vi "FPGAcode4_Debug.vi"(7 "Speed Bracket":i32, 8 "Thresholds in":i32[](array[numeric])=[0, 0, 0, 0, 0, 0, 0, 0, 0, 0, 0], 9 "Clock Speed (Hz)":i32=40000000, 10 "Calibrate":bool=TRUE, 11 "Detector Waveform In":sgl[][](array[numeric])) -> (0 "Thresholds out":i32[](array[numeric]), 1 "Charge":fxp<+,32,-41>[](array[numeric]), 2 "Mass":fxp<+/-,64,-19>[](array[numeric]), 3 "PSU Response":bool[](array[boolean]), 4 "Velocity Count":i32[](array[numeric]), 5 "Max Stop Point":T1)   [LabVIEW 2015]
uses:
  FPGA3/Limits_In.ctl
  FPGA3/Detector_Cluster.ctl
  FPGA3/Correlations.ctl
panel:
  in  "User Trigger?":bool
  in  "User Trigger Distance":fxp<+/-,34,18> format="%.3g"
  out "User Trigger":bool
  in  "Boxcar 3 Size Factor":fxp<+/-,32,16>=0.199951171875 format="%.2g"
  in  "Charge Error Factor":fxp<+/-,32,16>=1.499969482421875 format="%.2g"
  in  "Max Correlation Factor":fxp<+,32,4>=1.1000000052154064 format="%.3g"
  in  "Threshold Factor":fxp<+/-,32,16>=1.299957275390625 format="%.2g"
  out "DCS 2":bool
  out "DCS 1":bool
  in  "Limits":T2={"High Charge Limit"=4.54747350780585e-13, "Low Charge Limit"=0.0, "High Velocity Limit"=262143.0, "Low Velocity Limit"=0.0, "High Mass Limit"=7.27595761248936e-12, "Low Mass Limit"=0.0, "High Voltage"=2200000.0}
  in  "Armed":bool
  out "Plates":bool
  in  "One Shot":bool
  # "These factors above are in the front\npanel so it is possible to experiment\nwith many different configurations\nof the FPGA on the fly. One can even\nchange the relative size of one filter."
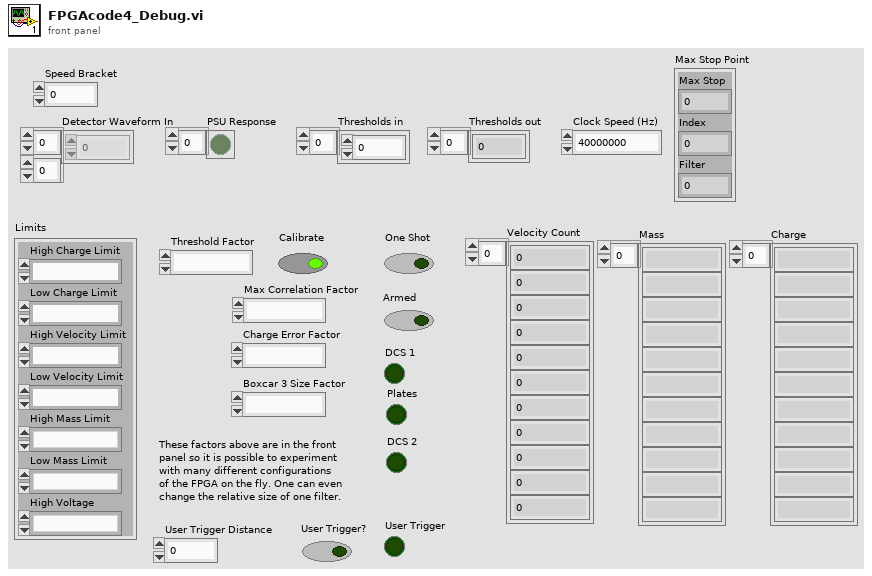
[diagram p1: front panel]
types:
  T1 = cluster{"Max Stop":u8, "Index":i32, "Filter":i32}
  T2 = typedef "Limits_In.ctl" = cluster{"High Charge Limit":fxp<+,32,-41>, "Low Charge Limit":fxp<+,32,-41>, "High Velocity Limit":fxp<+,18,18>, "Low Velocity Limit":fxp<+,18,18>, "High Mass Limit":fxp<+/-,33,-36>, "Low Mass Limit":fxp<+/-,33,-36>, "High Voltage":fxp<+,16,22>}
  T3 = cluster{i32, fxp<+/-,64,-19>, "High Charge Limit":fxp<+,32,-41>}[]
  T4 = typedef "Detector_Cluster.ctl" = cluster{"Det 1":i32, "Det 2":i32}
  T5 = cluster{"Filter 1":T4, "Filter 2":T4, "Filter 3":T4, "Filter 4":T4}
  T6 = cluster{"Distance to PSU":fxp<+/-,32,5>, "Distance to end of PSU":fxp<+/-,32,5>, "Distance to DCS 2":fxp<+/-,32,5>, "Distance to DCS 1":fxp<+/-,32,5>, "Distance to front of LEIL Chamber":fxp<+/-,32,5>}
  T7 = cluster{"Detector Max Speed Count":i32, "Detector Min Speed Count":i32, "Gap Max Speed Count":i32, "Gap Min Speed Count":i32}
  T8 = cluster{"Distance to PSU":fxp<+/-,64,37>, "Distance to end of PSU":fxp<+/-,64,37>, "Distance to DCS 2":fxp<+/-,64,37>, "Distance to DCS 1":fxp<+/-,64,37>, "Distance to front of LEIL Chamber":fxp<+/-,64,37>}
  T9 = cluster{"Filter 1":T4, "Filter 2":T4, "Filter 3":T4, "Filter 4":T4}[]
  T10 = cluster{"First Detector Count":i32, "Detector Gap Count":i32, "Second Detector Count":i32, "Second Detector Final Count":i32}
  T11 = typedef "Correlations.ctl" = cluster{"First Correlation":i32, "Latest Correlation":i32}
  T12 = cluster{cluster{i16, i16}, cluster{"Det 1":i16, "Det 2":i16}, cluster{"Det 1":i16, "Det 2":i16}, cluster{"Det 1":i16, "Det 2":i16}}
  T13 = cluster{cluster{"Det 1":i16, "Det 2":i16}, cluster{"Det 1":i16, "Det 2":i16}, cluster{"Det 1":i16, "Det 2":i16}, cluster{"Det 1":i16, "Det 2":i16}}
  T14 = cluster{"Distance to PSU":fxp<+/-,64,69>, "Distance to end of PSU":fxp<+/-,64,69>, "Distance to DCS 2":fxp<+/-,64,69>, "Distance to DCS 1":fxp<+/-,64,69>, "Distance to front of LEIL Chamber":fxp<+/-,64,69>}
  T15 = cluster{"Distance to PSU":i32, "Distance to end of PSU":i32, "Distance to DCS 2":i32, "Distance to DCS 1":i32, "Distance to front of LEIL Chamber":i32}
  T16 = cluster{i32, fxp<+/-,64,-19>, "High Charge Limit":fxp<+,32,-41>}
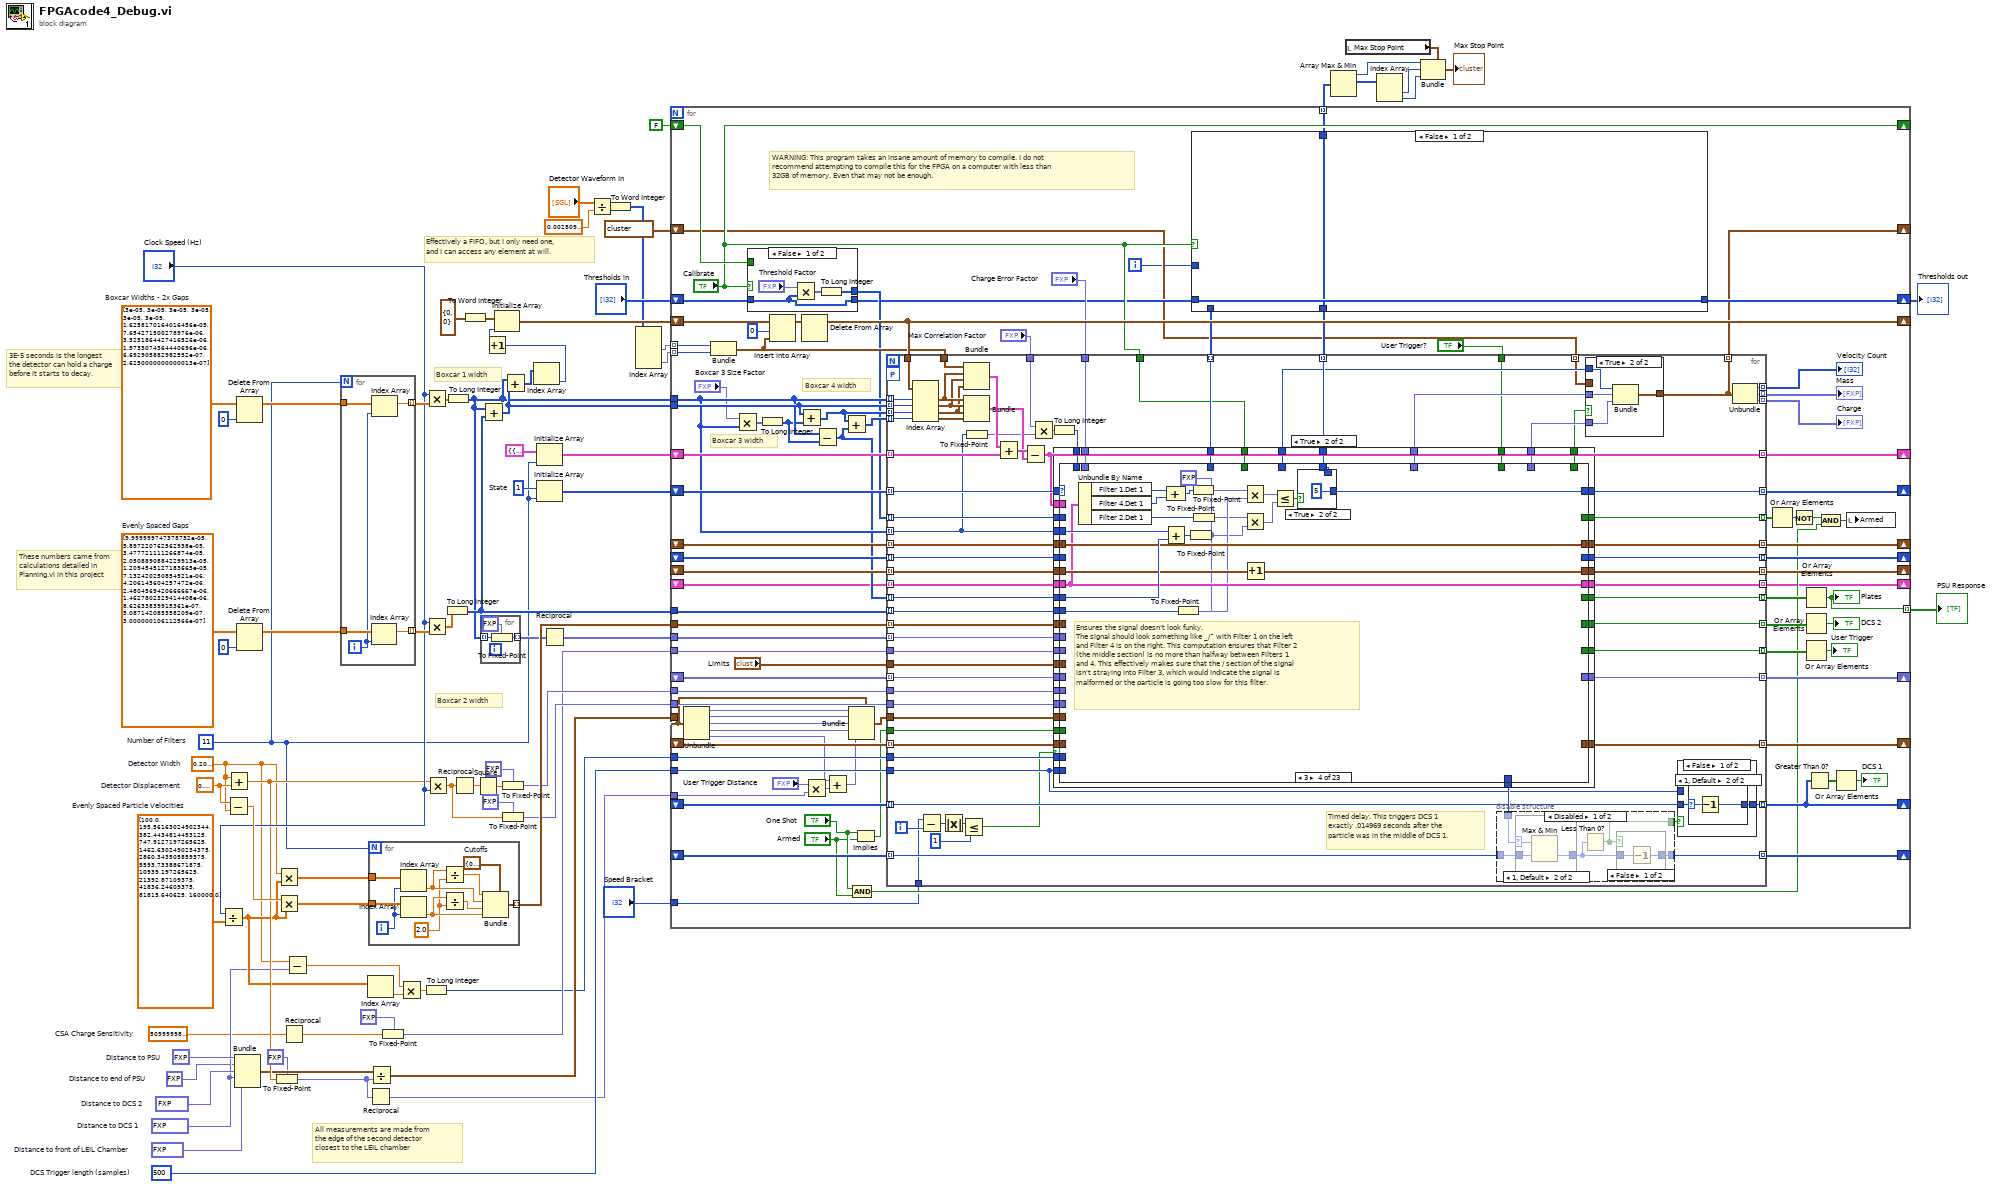
[diagram p0: block diagram]
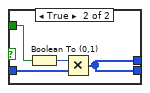
[diagram p2: hidden frame]
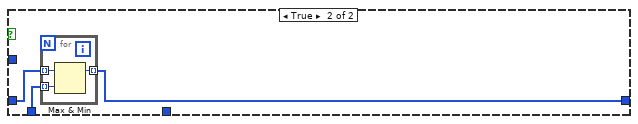
[diagram p3: hidden frame]
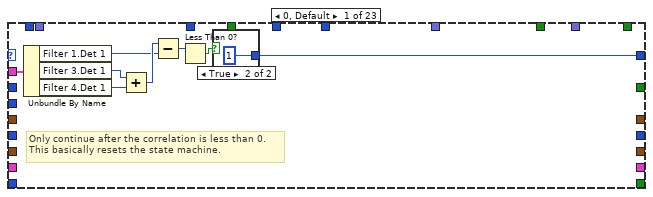
[diagram p5: hidden frame]
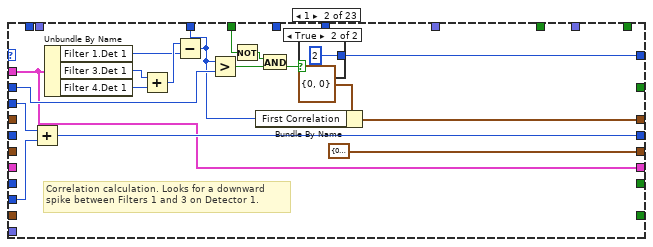
[diagram p7: hidden frame]
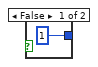
[diagram p8: hidden frame]
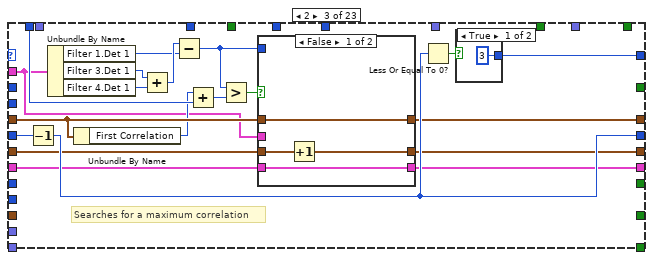
[diagram p9: hidden frame]
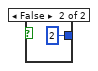
[diagram p10: hidden frame]
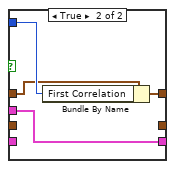
[diagram p11: hidden frame]
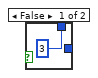
[diagram p12: hidden frame]
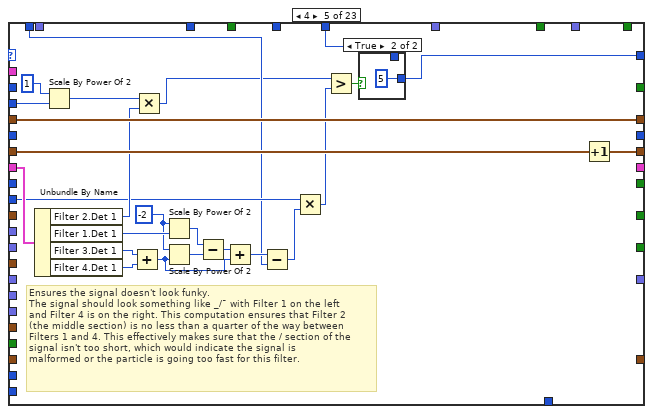
[diagram p13: hidden frame]
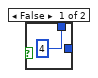
[diagram p14: hidden frame]
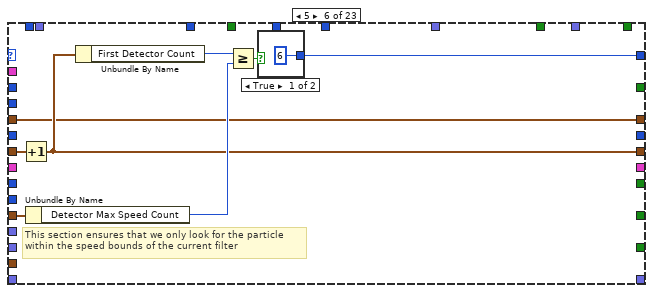
[diagram p15: hidden frame]
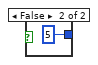
[diagram p16: hidden frame]
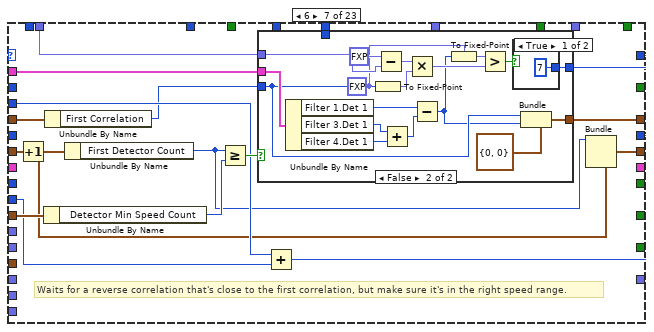
[diagram p17: hidden frame]
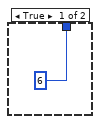
[diagram p18: hidden frame]
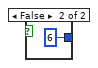
[diagram p19: hidden frame]
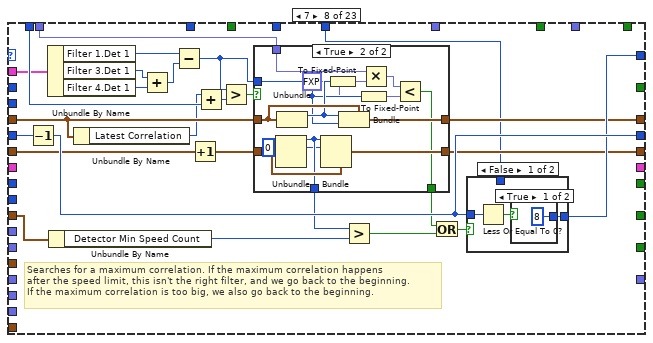
[diagram p20: hidden frame]
diagram:
  w10 = dbl[] [3e-05, 3e-05, 3e-05, 3e-05, 3e-05, 3e-05, 1.6258170164016456e-05, 7.654271500278976e-06, 3.5251864427416526e-06, 1.5733074364440696e-06, 6.692905882982552e-07, 2.6250000000000013e-07]  # Boxcar Widths - 2x Gaps
  w28 = fxp<+/-,32,5> 4.297679997980595  # Distance to front of LEIL Chamber
  w34 = u16 500  # DCS Trigger length (samples)
  w39 = fxp<+/-,32,5> -1.3589000031352043  # Distance to DCS 1
  w42 = fxp<+/-,32,5> 2.6162000000476837  # Distance to DCS 2
  w31 = fxp<+/-,32,5> 2.0  # Distance to end of PSU
  w43 = fxp<+/-,32,5> 1.1000000014901161  # Distance to PSU
  w27 = sgl 5100000000000000.0  # CSA Charge Sensitivity
  w74 = u8 1  # State
  w40 = sgl 0.6  # Detector Displacement
  w78 = sgl[] [0.0001, 5.8972208e-05, 3.477721e-05, 2.050889e-05, 1.2094545e-05, 7.1324203e-06, 4.2061456e-06, 2.480457e-06, 1.4627802e-06, 8.6263384e-07, 5.087142e-07, 3e-07]  # Evenly Spaced Gaps
  w59 = sgl[] [100.0, 195.56163, 382.44348, 747.9127, 1462.6302, 2860.3435, 5593.734, 10939.197, 21392.871, 41836.246, 81815.64, 160000.0]  # Evenly Spaced Particle Velocities
  w35 = sgl 0.21  # Detector Width
  w32 = 11  # Number of Filters
  # "All measurements are made from\nthe edge of the second detector\nclosest to the LEIL chamber"
  # "Effectively a FIFO, but I only need one,\nand I can access any element at will."
  # "Boxcar 2 width"
  # "Boxcar 1 width"
  # "3E-5 seconds is the longest\nthe detector can hold a charge\nbefore it starts to decay."
  # "These numbers came from\ncalculations detailed in\nPlanning.vi in this project"
  n1 = Divide(x="Clock Speed (Hz)", y=w59) -> (x/y=w41:sgl[])
  n2 = Subtract(x=w40, y=w35) -> (x-y=w58:sgl)
  n3 = Add(x=w35, y=w40) -> (x+y=w46:sgl)
  n4 = Bundle("Distance to PSU"=w43, "Distance to end of PSU"=w31, "Distance to DCS 2"=w42, "Distance to DCS 1"=w39, "Distance to front of LEIL Chamber"=w28) -> (w45:T6)  [unwired: 1 in]
  n5 = Delete From Array(array=w10, index=0) -> (array with subset deleted=w67:dbl[])  [unwired: 1 in, 1 out]
  n6 = Delete From Array(array=w78, index=0) -> (array with subset deleted=w69:sgl[])  [unwired: 1 in, 1 out]
  n7 = To Fixed-Point(fixed-point type=fxp<+/-,32,1> 0.0, number=w46) -> (fixed-point=w30:fxp<+/-,32,1>)
  n8 = Multiply(x=w35, y=w41) -> (x*y=w76:sgl[])
  n9 = Multiply(x=w58, y=w41) -> (x*y=w77:sgl[])
  n10 = Reciprocal(x=w27) -> (1/x=w48:sgl)
  n11 = Subtract(x=w35, y=w39) -> (x-y=w37:sgl)
  n12 = for {
    N: w32 -> [_]
    tunnel: w69 -> [w86]
    tunnel: [w83] -> w68 mode=indexing
    tunnel: w67 -> [w85]
    tunnel: [w84] -> w66 mode=indexing
    i -> [w82]
    n13 = Index Array(array=w86, index=w82) -> (element=w83:sgl)
    n14 = Index Array(array=w85, index=w82) -> (element=w84:dbl)
  }
  n15 = Index Array(array=w41) -> (element=w38:sgl)  [unwired: 1 in]
  n16 = Reciprocal(x=w30) -> (1/x=w29:fxp<+/-,34,33>)
  n17 = for {
    N: w32 -> [_]
    tunnel: w77 -> [w96]
    tunnel: w76 -> [w95]
    tunnel: [w94] -> w71 mode=indexing
    i -> [w93]
    w87 = sgl 2.0 ("y")
    w92 = T7 {"Detector Max Speed Count"=0, "Detector Min Speed Count"=0, "Gap Max Speed Count"=0, "Gap Min Speed Count"=0}  # Cutoffs
    n18 = Index Array(array=w95, index=w93) -> (element=w91:sgl)
    n19 = Index Array(array=w96, index=w93) -> (element=w88:sgl)
    n20 = Divide(x=w91, y=w87) -> (x/y=w90:sgl)
    n21 = Divide(x=w88, y=w87) -> (x/y=w89:sgl)
    n22 = Bundle(cluster=w92, "Detector Max Speed Count"=w90, "Detector Min Speed Count"=w91, "Gap Max Speed Count"=w89, "Gap Min Speed Count"=w88) -> (w94:T7)
  }
  n23 = Divide(x=w45, y=w30) -> (x/y=w44:T8)
  n24 = To Fixed-Point(fixed-point type=fxp<+,32,-51> 0.0, number=w48) -> (fixed-point=w47:fxp<+,32,-51>)
  n25 = Multiply(x=w37, y=w38) -> (x*y=w36:sgl)
  n26 = To Long Integer(number=w36) -> (32bit integer=w33:i32)
  n27 = Multiply(x="Clock Speed (Hz)", y=w66) -> (x*y=w70:dbl[])
  n28 = Multiply(x="Clock Speed (Hz)", y=w68) -> (x*y=w75:sgl[])
  n29 = Multiply(x=w46, y="Clock Speed (Hz)") -> (x*y=w51:sgl)
  n30 = To Long Integer(number=w75) -> (32bit integer=w65:i32[])
  n31 = To Long Integer(number=w70) -> (32bit integer=w22:i32[])
  n32 = Reciprocal(x=w51) -> (1/x=w55:sgl)
  n33 = To Word Integer(number=T4 {"Det 1"=0, "Det 2"=0} ("Detectors")) -> (16bit integer=w64:cluster{"Det 1":i16, "Det 2":i16})
  n34 = Square(x=w55) -> (x^2=w54:sgl)
  n35 = Add(x=w22, y=w65) -> (x+y=w23:i32[])
  n36 = for {
    tunnel: w22 -> [w99] mode=indexing
    tunnel: [w98] -> w61 mode=indexing
    n37 = To Fixed-Point(fixed-point type=fxp<+/-,32,32> 0.0, number=w99) -> (fixed-point=w98:fxp<+/-,32,32>)
  }
  n38 = To Fixed-Point(fixed-point type=fxp<+/-,32,-42> 0.0, number=w54) -> (fixed-point=w57:fxp<+/-,32,-42>)
  n39 = To Fixed-Point(fixed-point type=fxp<+,32,28> 0.0, number=w51) -> (fixed-point=w49:fxp<+,32,28>)
  n40 = Add(x=w22, y=w23) -> (x+y=w21:i32[])
  n41 = Index Array(array=w21) -> (element=w20:i32)  [unwired: 1 in]
  n42 = Increment(x=w20) -> (x+1=w19:i32)
  n43 = Initialize Array(w64, w19) -> (w81:cluster{"Det 1":i16, "Det 2":i16}[])
  n44 = Initialize Array(T5 {"Filter 1"={"Det 1"=0, "Det 2"=0}, "Filter 2"={"Det 1"=0, "Det 2"=0}, "Filter 3"={"Det 1"=0, "Det 2"=0}, "Filter 4"={"Det 1"=0, "Det 2"=0}} ("cluster"), w32) -> (w72:T9)
  n45 = Initialize Array(w74, w32) -> (w73:u8[])
  n46 = Reciprocal(x=w61) -> (1/x=w60:fxp<+/-,34,2>[])
  n47 = Divide(x="Detector Waveform In", y=sgl 0.00281) -> (x/y=w26:sgl[][])
  n48 = To Word Integer(number=w26) -> (16bit integer=w12:i16[][])
  n49 = Index Array(array=w12) -> (element #1=w14:i16[], element #2=w13:i16[])  [unwired: 4 in]
  n50 = for {
    shift-right: [w188] -> _
    shift-left: w81 -> [w189]
    shift-right: [w187] -> _
    shift-left: w72 -> [w180]
    shift-right: [w185] -> _
    shift-left: w73 -> [w186]
    shift-right: [w184] -> _
    shift-left: _ -> [w183]
    shift-right: [w182] -> _
    shift-left: _ -> [w181]
    tunnel: w71 -> [w179]
    shift-right: [w178] -> _
    shift-left: _ -> [w177]
    tunnel: w22 -> [w174]
    tunnel: w23 -> [w176]
    tunnel: w65 -> [w175]
    tunnel: w60 -> [w173]
    shift-right: [w172] -> _
    shift-left: _ -> [w171]
    tunnel: w57 -> [w170]
    tunnel: w47 -> [w169]
    tunnel: w49 -> [w168]
    tunnel: w44 -> [w155]
    shift-right: [w167] -> _
    shift-left: _ -> [w166]
    shift-right: [w165] -> w24
    shift-left: "Thresholds in" -> [w164]
    shift-right: ["Calibrate"] -> _
    shift-left: FALSE ("Calibrate") -> [w163]
    tunnel: w34 -> [w162]
    tunnel: w33 -> [w161]
    shift-right: [w159] -> _
    shift-left: _ -> [w160]
    shift-right: [w158] -> _
    shift-left: _ -> [w157]
    tunnel: w29 -> [w156]
    shift-right: [w107] -> _
    shift-left: T3 [{0, 0.0, "High Charge Limit"=0.0}, {0, 0.0, "High Charge Limit"=0.0}, {0, 0.0, "High Charge Limit"=0.0}, {0, 0.0, "High Charge Limit"=0.0}, {0, 0.0, "High Charge Limit"=0.0}, {0, 0.0, "High Charge Limit"=0.0}, {0, 0.0, "High Charge Limit"=0.0}, {0, 0.0, "High Charge Limit"=0.0}, {0, 0.0, "High Charge Limit"=0.0}, {0, 0.0, "High Charge Limit"=0.0}, {0, 0.0, "High Charge Limit"=0.0}] -> [w106]
    tunnel: [w115] -> w9 mode=indexing
    shift-right: [w114] -> _
    shift-left: _ -> [w113]
    tunnel: w14 -> [w112] mode=indexing
    tunnel: w13 -> [w111] mode=indexing
    tunnel: [w102] -> w8 mode=indexing
    tunnel: "Speed Bracket" -> [w100]
    i -> [w101]
    # "WARNING: This program takes an insane amount of memory to compile. I do not\nrecommend attempting to compile this for the FPGA on a computer with less than\n32GB of memory. Even that may not be enough."
    # "Boxcar 3 width"
    # "Boxcar 4 width"
    n51 = Unbundle(w155) -> ("Distance to PSU"=w137:fxp<+/-,64,37>, "Distance to end of PSU"=w136:fxp<+/-,64,37>, "Distance to DCS 2"=w135:fxp<+/-,64,37>, "Distance to DCS 1"=w132:fxp<+/-,64,37>, "Distance to front of LEIL Chamber"=w131:fxp<+/-,64,37>)
    n52 = Bundle(w112, w111) -> (w116:cluster{i16, i16})  [unwired: 1 in]
    n53 = Multiply(x="Boxcar 3 Size Factor", y=w174) -> (x*y=w150:fxp<+/-,64,48>[])
    n54 = case shown="False" "Calibrate" {
      tunnel: w164 -> [w191 w197]
      tunnel: [w191 w194] -> w108
      tunnel: w163 -> [_ w196]
      tunnel: [w190 w194] -> w109
      frame False {
        n55 = Multiply(x="Threshold Factor", y=w191) -> (x*y=w192:fxp<+/-,64,48>[])
        n56 = To Long Integer(number=w192) -> (32bit integer=w190:i32[])
      }
      frame True {
        n57 = Boolean To (0,1)(Boolean=w196) -> (0, 1=w195:i16)
        n58 = Multiply(x=w195, y=w197) -> (x*y=w194:i32[])
      }
    }
    n59 = To Long Integer(number=w150) -> (32bit integer=w151:i32[])
    n60 = Insert Into Array(array=w189, index=0, new element=w116) -> (w154:cluster{"Det 1":i16, "Det 2":i16}[])
    n61 = Add(x=w176, y=w151) -> (x+y=w148:i32[])
    n62 = Delete From Array(array=w154) -> (array with subset deleted=w188:cluster{"Det 1":i16, "Det 2":i16}[])  [unwired: 2 in, 1 out]
    n63 = Multiply(x="User Trigger Distance", y=w156) -> (x*y=w133:fxp<+/-,64,49>)
    n64 = Subtract(x=w174, y=w151) -> (x-y=w146:i32[])
    n65 = Add(x=w131, y=w133) -> (x+y=w130:fxp<+/-,64,50>)
    n66 = Add(x=w148, y=w146) -> (x+y=w147:i32[])
    n67 = Bundle(cluster=w155, "Distance to PSU"=w137, "Distance to end of PSU"=w136, "Distance to DCS 2"=w135, "Distance to DCS 1"=w132, "Distance to front of LEIL Chamber"=w130) -> (w134:T8)
    n68 = And(x="One Shot", y="Armed") -> (x .and. y?=w121:bool)
    n69 = Implies(1:"Armed", 2:"One Shot") -> (0:w141:bool)
    n70 = for {
      tunnel: w188 -> [w282]
      tunnel: [w265] -> w187 mode=indexing
      tunnel: w186 -> [w281] mode=indexing
      tunnel: [w279] -> w185 mode=indexing
      tunnel: w109 -> [w280] mode=indexing
      tunnel: [w278] -> w184 mode=indexing
      tunnel: w183 -> [w277] mode=indexing
      tunnel: [w276] -> w182 mode=indexing
      tunnel: w181 -> [w275] mode=indexing
      tunnel: w180 -> [w269] mode=indexing
      tunnel: w116 -> [w274]
      tunnel: w179 -> [w264] mode=indexing
      tunnel: [w263] -> w178 mode=indexing
      tunnel: w177 -> [w262] mode=indexing
      tunnel: w174 -> [w261] mode=indexing
      tunnel: w176 -> [w260] mode=indexing
      tunnel: w148 -> [w259] mode=indexing
      tunnel: w147 -> [w258] mode=indexing
      tunnel: w174 -> [w207] mode=indexing
      tunnel: "Max Correlation Factor" -> [w257]
      tunnel: w146 -> [w256] mode=indexing
      tunnel: w175 -> [w206] mode=indexing
      tunnel: "Charge Error Factor" -> [w255]
      tunnel: [w254] -> w143 mode=indexing
      tunnel: w173 -> [w253] mode=indexing
      tunnel: "Limits" -> [w252]
      tunnel: [w251] -> w172 mode=indexing
      tunnel: w171 -> [w250] mode=indexing
      tunnel: w170 -> [w249]
      tunnel: w169 -> [w248]
      tunnel: w168 -> [w247]
      tunnel: w134 -> [w246]
      tunnel: [w245] -> w167 mode=indexing
      tunnel: w166 -> [w244] mode=indexing
      tunnel: [w243] -> w142 mode=indexing
      tunnel: w141 -> [w242]
      tunnel: w162 -> [w239]
      tunnel: w161 -> [w241]
      tunnel: [w238] -> w159 mode=indexing
      tunnel: w160 -> [w237] mode=indexing
      tunnel: [w235] -> w158 mode=indexing
      tunnel: w157 -> [w234] mode=indexing
      tunnel: [w233] -> w129 mode=indexing
      tunnel: [w232] -> w128 mode=indexing
      tunnel: [w231] -> w127 mode=indexing
      tunnel: [w230] -> w124 mode=indexing
      tunnel: "User Trigger?" -> [w223]
      tunnel: w113 -> [w220] mode=indexing
      tunnel: [w219] -> w114 mode=indexing
      tunnel: "Calibrate" -> [w217]
      tunnel: [w215] -> w107 mode=indexing
      tunnel: w106 -> [w216] mode=indexing
      tunnel: [w214] -> w105 mode=indexing
      tunnel: [w213] -> w104 mode=indexing
      tunnel: [w212] -> w103 mode=indexing
      workers-P: _ -> [_]
      tunnel: w100 -> [w211]
      i -> [w222]
      # "Timed delay. This triggers DCS 1\nexactly .014969 seconds after the\nparticle was in the middle of DCS 1."
      n71 = Index Array(array=w282, index #1=w261, index #2=w260, index #3=w259, index #4=w258) -> (element #1=w272:cluster{"Det 1":i16, "Det 2":i16}, element #2=w271:cluster{"Det 1":i16, "Det 2":i16}, element #3=w270:cluster{"Det 1":i16, "Det 2":i16}, element #4=w273:cluster{"Det 1":i16, "Det 2":i16})
      n72 = Subtract(x=w211, y=w222) -> (x-y=w221:i32)
      n73 = Absolute Value(x=w221) -> (abs(x)=w210:i32)
      n74 = Less Or Equal?(x=w210, y=1) -> (x <= y?=w209:bool)
      n75 = Bundle(w274, w272, w271, w270) -> (w268:T12)  [unwired: 1 in]
      n76 = Bundle(w272, w271, w270, w273) -> (w266:T13)  [unwired: 1 in]
      n77 = To Fixed-Point(number=w207) -> (fixed-point=w225:fxp<+/-,32,32>)  [unwired: 1 in]
      n78 = Add(x=w268, y=w269) -> (x+y=w267:T5)
      n79 = Subtract(x=w267, y=w266) -> (x-y=w265:T5)
      n80 = Multiply(x=w257, y=w225) -> (x*y=w226:fxp<+/-,64,36>)
      n81 = To Long Integer(number=w226) -> (32bit integer=w224:i32)
      n82 = case shown="True" w209 {
        tunnel: w281 -> [_ w326]
        tunnel: w280 -> [_ w325]
        tunnel: [_ w324] -> w279
        tunnel: [_ w323] -> w278
        tunnel: w277 -> [_ w322]
        tunnel: [_ w321] -> w276
        tunnel: w275 -> [_ w320]
        tunnel: w265 -> [_ w319]
        tunnel: w264 -> [_ w318]
        tunnel: [_ w317] -> w263
        tunnel: w262 -> [_ w316]
        tunnel: w256 -> [_ w315]
        tunnel: w206 -> [_ w314]
        tunnel: w255 -> [_ w313]
        tunnel: [_ w312] -> w254
        tunnel: w253 -> [_ w311]
        tunnel: w252 -> [_ w310]
        tunnel: [_ w309] -> w251
        tunnel: w250 -> [_ w308]
        tunnel: w249 -> [_ w307]
        tunnel: w248 -> [_ w306]
        tunnel: w247 -> [_ w305]
        tunnel: w246 -> [_ w304]
        tunnel: [_ w303] -> w245
        tunnel: w244 -> [_ w302]
        tunnel: [_ w301] -> w243
        tunnel: w242 -> [_ w300]
        tunnel: w241 -> [_ w299]
        tunnel: [_ w298] -> w240
        tunnel: w239 -> [_ w297]
        tunnel: [_ w296] -> w233
        tunnel: [_ w295] -> w232
        tunnel: [_ w294] -> w231
        tunnel: [_ w293] -> w230
        tunnel: [_ w292] -> w229
        tunnel: [_ w291] -> w228
        tunnel: [_ w290] -> w227
        tunnel: w207 -> [_ w289]
        tunnel: w224 -> [_ w288]
        tunnel: w223 -> [_ w287]
        tunnel: [_ w286] -> w219
        tunnel: w220 -> [_ w285]
        tunnel: [_ w284] -> w218
        tunnel: w217 -> [_ w283]
        frame False {
        }
        frame True {
          n83 = case shown="3" w326 {
            tunnel: w325 -> [_ w353 _ _ _ _ _ _ _ _ _ _ _ _ _ _ _ _ _ _ _ _ _]
            tunnel: [w333 w351 w371 w406 w434 w439 w453 w506 w549 w562 w581 w635 w664 w687 w739 w785 u8 17 ("Det 3") w823 w831 w838 w852 w858 w871] -> w324
            tunnel: w289 -> [_ w344 _ w404 w417 _ w456 _ _ _ w584 _ _ w690 _ _ w813 _ _ _ _ _ _]
            tunnel: [_ w346 w367 w405 w433 w437 w450 w504 w545 w568 w578 w633 w670 w684 w737 _ _ _ _ _ _ _ _] -> w323
            tunnel: w322 -> [_ _ w366 w405 w433 w437 w452 w503 w544 w568 w580 w632 w670 w686 w736 _ _ _ _ _ _ _ _]
            tunnel: [_ w343 w373 _ _ _ w454 w508 _ _ w582 w637 _ w688 w741 _ _ _ _ _ _ _ _] -> w321
            tunnel: w320 -> [_ _ w375 _ _ _ _ w510 _ _ _ w639 _ _ w743 _ _ _ _ _ _ _ _]
            tunnel: w319 -> [w328 w340 w357 _ _ _ w457 w485 _ _ w585 w630 _ w680 w734 _ _ _ _ _ _ _ _]
            tunnel: w318 -> [_ _ _ _ _ w444 w462 w495 _ w567 w590 w623 w669 w694 w727 _ _ _ _ _ _ _ _]
            tunnel: [_ T10 {"First Detector Count"=0, "Detector Gap Count"=0, "Second Detector Count"=0, "Second Detector Final Count"=0} ("Cutoffs") w361 w402 w431 w438 w448 w499 w547 w566 w576 w627 w668 w678 w731 w800 _ _ _ _ _ _ _] -> w317
            tunnel: w316 -> [_ _ w372 w403 w432 w443 w463 w507 w548 w569 w591 w636 w671 w695 w740 w801 w821 _ _ _ _ _ _]
            tunnel: w288 -> [_ _ w374 _ w412 _ _ w509 _ _ _ w638 _ _ w742 _ _ _ _ _ _ _ _]
            tunnel: w315 -> [_ _ _ w407 _ _ _ _ _ _ _ _ _ _ _ _ _ _ _ _ _ _ _]
            tunnel: w314 -> [_ w342 _ w396 w416 _ w455 _ _ _ w583 _ _ w689 _ _ _ _ _ _ _ _ _]
            tunnel: w313 -> [_ _ _ _ _ _ w458 w487 _ _ w586 w615 _ w691 w720 _ _ _ _ _ _ _ _]
            tunnel: [_ _ _ w401 w430 _ w459 w489 w550 _ w587 w617 _ w692 w722 w784 _ _ _ _ _ _ _] -> w312
            tunnel: w311 -> [_ _ _ _ _ _ _ _ w555 _ _ _ _ _ _ _ _ _ _ _ _ _ _]
            tunnel: w310 -> [_ _ _ _ _ _ _ _ w558 _ _ _ _ _ _ w802 _ _ _ _ _ _ _]
            tunnel: [_ _ _ _ _ _ _ _ w534 w561 w573 w613 w663 w682 w718 _ _ _ _ _ _ _ _] -> w309
            tunnel: w308 -> [_ _ _ _ _ _ _ _ _ w561 w573 w613 w663 w682 w718 w768 _ _ _ _ _ _ _]
            tunnel: w307 -> [_ _ _ _ _ _ _ _ _ _ _ _ _ _ _ w796 _ _ _ _ _ _ _]
            tunnel: w306 -> [_ _ _ _ _ _ _ _ w542 _ _ _ _ _ _ _ _ _ _ _ _ _ _]
            tunnel: w305 -> [_ _ _ _ _ _ _ _ _ _ _ _ _ _ _ w778 _ _ _ _ _ _ _]
            tunnel: w304 -> [_ _ _ _ _ _ _ _ _ _ _ _ _ _ _ _ w817 _ _ _ _ _ _]
            tunnel: [_ _ _ _ _ _ _ _ _ _ _ _ _ _ _ _ w809 w825 w833 w840 w849 w860 w869] -> w303
            tunnel: w302 -> [_ _ _ _ _ _ _ _ _ _ _ _ _ _ _ _ _ w826 w834 w841 w850 w861 w870]
            tunnel: [_ w339 _ _ _ _ _ _ _ _ _ _ _ _ _ _ _ _ _ _ _ _ _] -> w301
            tunnel: w300 -> [_ _ _ _ _ _ _ _ _ _ _ _ _ _ _ w777 _ _ _ _ _ _ _]
            tunnel: w299 -> [_ _ _ _ _ _ _ _ _ _ _ _ _ _ _ _ w808 _ _ _ _ _ _]
            tunnel: w297 -> [_ _ _ _ _ _ _ _ _ _ _ _ _ _ _ _ _ _ _ _ w847 _ w867]
            tunnel: [_ _ _ _ _ _ _ _ _ _ _ _ _ _ _ _ w806 _ _ _ _ _ _] -> w298
            tunnel: [_ _ _ _ _ _ _ _ _ _ _ _ _ _ _ _ _ _ TRUE _ _ _ _] -> w296
            tunnel: [_ _ _ _ _ _ _ _ _ _ _ _ _ _ _ _ _ _ _ _ TRUE _ _] -> w295
            tunnel: [_ _ _ _ _ _ _ _ _ _ _ _ _ _ _ _ _ _ _ _ _ _ TRUE] -> w294
            tunnel: [_ _ _ _ _ _ _ _ _ _ _ _ _ _ _ w776 _ _ _ _ _ _ _] -> w293
            tunnel: [_ _ _ _ _ _ _ _ _ _ _ _ _ _ _ w769 _ _ _ _ _ _ _] -> w290
            tunnel: [_ _ _ _ _ _ _ _ _ _ _ _ _ _ _ w768 _ _ _ _ _ _ _] -> w292
            tunnel: [_ _ _ _ _ _ _ _ _ _ _ _ _ _ _ w773 _ _ _ _ _ _ _] -> w291
            tunnel: w287 -> [_ _ _ _ _ _ _ _ _ _ _ _ _ _ _ _ _ _ _ _ w844 _ _]
            tunnel: [_ w340 w358 w391 _ _ _ _ _ _ _ _ _ _ _ _ _ _ _ _ _ _ _] -> w286
            tunnel: w285 -> [_ _ w356 w391 w429 _ _ _ _ _ _ _ _ _ _ _ _ _ _ _ _ _ _]
            tunnel: [_ _ _ _ _ _ _ _ _ _ _ _ _ _ _ TRUE ("result") _ _ _ _ _ _ _] -> w284
            tunnel: w283 -> [_ w336 _ _ _ _ _ _ _ _ _ _ _ _ _ _ _ _ _ _ _ _ _]
            frame 0, Default {
              # "Only continue after the correlation is less than 0.\nThis basically resets the state machine."
              n84 = Unbundle By Name(w328) -> ("Filter 1.Det 1"=w329:i32, "Filter 3.Det 1"=w330:i32, "Filter 4.Det 1"=w331:i32)
              n85 = Add(x=w330, y=w331) -> (x+y=w332:i32)
              n86 = Subtract(x=w332, y=w329) -> (x-y=w327:i32)
              n87 = Less Than 0?(x=w327) -> (x < 0?=w334:bool)
              n88 = case shown="True" w334 {
                tunnel: [_ u8 1 ("Det 3")] -> w333
                frame False {
                }
                frame True {
                }
              }
            }
            frame 1 {
              # "Correlation calculation. Looks for a downward\nspike between Filters 1 and 3 on Detector 1."
              n89 = Add(x=w344, y=w342) -> (x+y=w343:i32)
              n90 = Unbundle By Name(w340) -> ("Filter 1.Det 1"=w347:i32, "Filter 3.Det 1"=w348:i32, "Filter 4.Det 1"=w349:i32)
              n91 = Add(x=w348, y=w349) -> (x+y=w350:i32)
              n92 = Subtract(x=w350, y=w347) -> (x-y=w339:i32)
              n93 = Greater?(x=w339, y=w353) -> (0:w352:bool)
              n94 = Not(x=w336) -> (.not. x?=w337:bool)
              n95 = Bundle By Name(cluster=T11 {"First Correlation"=0, "Latest Correlation"=0}, "First Correlation"=w339) -> (w346:T11)
              n96 = And(x=w337, y=w352) -> (x .and. y?=w338:bool)
              n97 = case shown="True" w338 {
                tunnel: [u8 1 ("Det 3") u8 2 ("Det 3")] -> w351
                frame False {
                }
                frame True {
                }
              }
            }
            frame 2 {
              # "Searches for a maximum correlation"
              n98 = Decrement(x=w375) -> (x-1=w373:i32)
              n99 = Unbundle By Name(w357) -> ("Filter 1.Det 1"=w364:i32, "Filter 3.Det 1"=w363:i32, "Filter 4.Det 1"=w362:i32)
              n100 = Unbundle By Name(w366) -> ("First Correlation"=w359:i32)
              n101 = Add(x=w363, y=w362) -> (x+y=w370:i32)
              n102 = Subtract(x=w370, y=w364) -> (x-y=w365:i32)
              n103 = Add(x=w359, y=w374) -> (x+y=w360:i32)
              n104 = Greater?(x=w365, y=w360) -> (0:w369:bool)
              n105 = case shown="False" w369 {
                tunnel: [w379 _] -> w361
                tunnel: w372 -> [w380 _]
                tunnel: w365 -> [_ w385]
                tunnel: [w381 w384] -> w367
                tunnel: w366 -> [w381 w383]
                tunnel: [w378 w382] -> w358
                tunnel: w357 -> [_ w382]
                tunnel: w356 -> [w378 _]
                frame False {
                  n106 = Increment(x=w380) -> (x+1=w379:T10)
                }
                frame True {
                  n107 = Bundle By Name(cluster=w383, "First Correlation"=w385) -> (w384:T11)
                }
              }
              n108 = Less Or Equal To 0?(x=w373) -> (x <= 0?=w368:bool)
              n109 = case shown="True" w368 {
                tunnel: [u8 3 ("Det 3") u8 2 ("Det 3")] -> w371
                frame True {
                }
                frame False {
                }
              }
            }
            frame 3 {
              w386 = fxp<+/-,32,32> 0.0 ("fixed-point type")
              # "Ensures the signal doesn't look funky.\nThe signal should look something like _/¯ with Filter 1 on the left\nand Filter 4 is on the right. This computation ensures that Filter 2\n(the middle section) is no more than halfway between Filters 1\nand 4. This effectively makes sure that the / section of the signal\nisn't straying into Filter 3, which would indicate the signal is\nmalformed or the particle is going too slow for this filter."
              n110 = Unbundle By Name(w391) -> ("Filter 1.Det 1"=w399:i32, "Filter 4.Det 1"=w400:i32, "Filter 2.Det 1"=w398:i32)
              n111 = Add(x=w404, y=w407) -> (x+y=w392:i32)
              n112 = Compound Arithmetic op=ADD(w399, w400) -> (w393:i32)
              n113 = To Fixed-Point(fixed-point type=w386, number=w396) -> (fixed-point=w389:fxp<+/-,32,32>)
              n114 = To Fixed-Point(fixed-point type=w386, number=w392) -> (fixed-point=w388:fxp<+/-,32,32>)
              n115 = To Fixed-Point(fixed-point type=w386, number=w393) -> (fixed-point=w390:fxp<+/-,32,32>)
              n116 = To Fixed-Point(fixed-point type=w386, number=w398) -> (fixed-point=w387:fxp<+/-,32,32>)
              n117 = Multiply(x=w390, y=w389) -> (x*y=w394:fxp<+/-,64,64>)
              n118 = Multiply(x=w387, y=w388) -> (x*y=w395:fxp<+/-,64,64>)
              n119 = Increment(x=w403) -> (x+1=w402:T10)
              n120 = Less Or Equal?(x=w394, y=w395) -> (x <= y?=w397:bool)
              n121 = case shown="True" w397 {
                tunnel: [_ u8 5] -> w406
                tunnel: [u8 3 _] -> w401
                frame False {
                }
                frame True {
                }
              }
            }
            frame 4 {
              w425 = i16 -2 ("n")
              # "Ensures the signal doesn't look funky.\nThe signal should look something like _/¯ with Filter 1 on the left\nand Filter 4 is on the right. This computation ensures that Filter 2\n(the middle section) is no less than a quarter of the way between\nFilters 1 and 4. This effectively makes sure that the / section of the\nsignal isn't too short, which would indicate the signal is\nmalformed or the particle is going too fast for this filter."
              n122 = Unbundle By Name(w429) -> ("Filter 2.Det 1"=w418:i32, "Filter 1.Det 1"=w426:i32, "Filter 3.Det 1"=w428:i32, "Filter 4.Det 1"=w427:i32)
              n123 = Scale By Power Of 2(n=i16 1, x=w417) -> (x*2^n=w419:i32)
              n124 = Add(x=w428, y=w427) -> (x+y=w421:i32)
              n125 = Multiply(x=w419, y=w418) -> (x*y=w410:i32)
              n126 = Scale By Power Of 2(n=w425, x=w426) -> (x*2^n=w424:i32)
              n127 = Scale By Power Of 2(n=w425, x=w421) -> (x*2^n=w423:i32)
              n128 = Subtract(x=w424, y=w423) -> (x-y=w422:i32)
              n129 = Add(x=w422, y=w421) -> (x+y=w414:i32)
              n130 = Subtract(x=w414, y=w412) -> (x-y=w413:i32)
              n131 = Multiply(x=w416, y=w413) -> (x*y=w411:i32)
              n132 = Greater?(x=w410, y=w411) -> (0:w415:bool)
              n133 = case shown="True" w415 {
                tunnel: [_ u8 5] -> w434
                tunnel: [u8 4 _] -> w430
                frame False {
                }
                frame True {
                }
              }
              n134 = Increment(x=w432) -> (x+1=w431:T10)
            }
            frame 5 {
              # "This section ensures that we only look for the particle\nwithin the speed bounds of the current filter"
              n135 = Increment(x=w443) -> (x+1=w438:T10)
              n136 = Unbundle By Name(w444) -> ("Detector Max Speed Count"=w441:i32)
              n137 = Unbundle By Name(w438) -> ("First Detector Count"=w442:i32)
              n138 = Greater Or Equal?(x=w442, y=w441) -> (x >= y?=w440:bool)
              n139 = case shown="True" w440 {
                tunnel: [u8 6 u8 5] -> w439
                frame True {
                }
                frame False {
                }
              }
            }
            frame 6 {
              # "Waits for a reverse correlation that's close to the first correlation, but make sure it's in the right speed range."
              n140 = Increment(x=w463) -> (x+1=w447:T10)
              n141 = Unbundle By Name(w462) -> ("Detector Min Speed Count"=w461:i32)
              n142 = Unbundle By Name(w452) -> ("First Correlation"=w451:i32)
              n143 = Unbundle By Name(w447) -> ("First Detector Count"=w449:i32)
              n144 = Greater Or Equal?(x=w449, y=w461) -> (x >= y?=w460:bool)
              n145 = case shown="False" w460 {
                tunnel: [_ w482] -> w453
                tunnel: [u8 6 _] -> w459
                tunnel: w458 -> [_ w481]
                tunnel: w457 -> [_ w478]
                tunnel: w451 -> [_ w468]
                tunnel: [_ w466] -> w450
                frame True {
                }
                frame False {
                  w465 = fxp<+/-,32,32> 0.0 ("fixed-point type")
                  n146 = Unbundle By Name(w478) -> ("Filter 1.Det 1"=w475:i32, "Filter 3.Det 1"=w477:i32, "Filter 4.Det 1"=w476:i32)
                  n147 = To Fixed-Point(fixed-point type=w465, number=w468) -> (fixed-point=w471:fxp<+/-,32,32>)
                  n148 = Subtract(x=fxp<+,1,2> 2.0, y=w481) -> (x-y=w479:fxp<+/-,33,17>)
                  n149 = Add(x=w477, y=w476) -> (x+y=w474:i32)
                  n150 = Multiply(x=w479, y=w471) -> (x*y=w473:fxp<+/-,64,48>)
                  n151 = Subtract(x=w475, y=w474) -> (x-y=w467:i32)
                  n152 = To Fixed-Point(fixed-point type=w465, number=w467) -> (fixed-point=w470:fxp<+/-,32,32>)
                  n153 = Greater?(x=w470, y=w473) -> (0:w472:bool)
                  n154 = case shown="True" w472 {
                    tunnel: [u8 7 u8 6] -> w482
                    frame True {
                    }
                    frame False {
                    }
                  }
                  n155 = Bundle(cluster=T11 {"First Correlation"=0, "Latest Correlation"=0} ("input cluster"), "First Correlation"=w468, "Latest Correlation"=w467) -> (w466:T11)
                }
              }
              n156 = Add(x=w456, y=w455) -> (x+y=w454:i32)
              n157 = Bundle(cluster=w447, "First Detector Count"=w449) -> (w448:T10)  [unwired: 3 in]
            }
            frame 7 {
              # "Searches for a maximum correlation. If the maximum correlation happens\nafter the speed limit, this isn't the right filter, and we go back to the beginning.\nIf the maximum correlation is too big, we also go back to the beginning."
              n158 = Decrement(x=w510) -> (x-1=w508:i32)
              n159 = Unbundle By Name(w485) -> ("Filter 1.Det 1"=w491:i32, "Filter 3.Det 1"=w501:i32, "Filter 4.Det 1"=w500:i32)
              n160 = Unbundle By Name(w495) -> ("Detector Min Speed Count"=w493:i32)
              n161 = Unbundle By Name(w503) -> ("Latest Correlation"=w497:i32)
              n162 = Add(x=w501, y=w500) -> (x+y=w490:i32)
              n163 = Subtract(x=w491, y=w490) -> (x-y=w502:i32)
              n164 = Increment(x=w507) -> (x+1=w496:T10)
              n165 = Add(x=w497, y=w509) -> (x+y=w498:i32)
              n166 = Greater?(x=w502, y=w498) -> (0:w505:bool)
              n167 = case shown="True" w505 {
                tunnel: [w517 w532] -> w499
                tunnel: w496 -> [w517 w529]
                tunnel: w502 -> [_ w523]
                tunnel: [w518 w531] -> w504
                tunnel: w503 -> [w518 w530]
                tunnel: [_ w528] -> w494
                tunnel: w487 -> [_ w527]
                tunnel: [_ w521] -> w486
                frame False {
                }
                frame True {
                  w520 = fxp<+/-,32,32> 0.0 ("fixed-point type")
                  n168 = Unbundle(w529) -> ("First Detector Count"=w528:i32)  [unwired: 3 out]
                  n169 = Unbundle(w530) -> ("First Correlation"=w526:i32)  [unwired: 1 out]
                  n170 = Bundle(cluster=w529, "First Detector Count"=w528, "Detector Gap Count"=0) -> (w532:T10)  [unwired: 2 in]
                  n171 = To Fixed-Point(fixed-point type=w520, number=w526) -> (fixed-point=w525:fxp<+/-,32,32>)
                  n172 = Bundle(cluster=w530, "First Correlation"=w526, "Latest Correlation"=w523) -> (w531:T11)
                  n173 = To Fixed-Point(fixed-point type=w520, number=w523) -> (fixed-point=w522:fxp<+/-,32,32>)
                  n174 = Multiply(x=w527, y=w525) -> (x*y=w524:fxp<+/-,64,48>)
                  n175 = Less?(x=w524, y=w522) -> (x < y?=w521:bool)
                }
              }
              n176 = Greater?(x=w494, y=w493) -> (0:w492:bool)
              n177 = Or(x=w486, y=w492) -> (x .or. y?=w488:bool)
              n178 = case shown="False" w488 {
                tunnel: w508 -> [w513 _]
                tunnel: [w512 _] -> w506
                tunnel: [_ u8 7 ("Det 3")] -> w489
                frame False {
                  n179 = Less Or Equal To 0?(x=w513) -> (x <= 0?=w511:bool)
                  n180 = case shown="True" w511 {
                    tunnel: [u8 8 ("Det 3") u8 7 ("Det 3")] -> w512
                    frame True {
                    }
                    frame False {
                    }
                  }
                }
                frame True {
                }
              }
            }
            frame 8 {
              # "q = ADC value / CSA sensitivity"
              # "Ensures the charge is good"
              n181 = Unbundle(w544) -> ("First Correlation"=w557:i32, "Latest Correlation"=w556:i32)
              n182 = Unbundle By Name(w558) -> ("High Charge Limit"=w533:fxp<+,32,-41>, "Low Charge Limit"=w554:fxp<+,32,-41>)
              n183 = Add(x=w557, y=w556) -> (x+y=w537:i32)
              n184 = Scale By Power Of 2(n=i16 -1, x=w537) -> (x*2^n=w535:i32)
              n185 = To Fixed-Point(fixed-point type=fxp<+/-,32,32> 0.0, number=w535) -> (fixed-point=w536:fxp<+/-,32,32>)
              n186 = Multiply(x=w536, y=w555) -> (x*y=w543:fxp<+/-,64,33>)
              n187 = Increment(x=w548) -> (x+1=w547:T10)
              n188 = To Long Integer(number=w535) -> (32bit integer=w546:i32)
              n189 = Multiply(x=w543, y=w542) -> (x*y=w541:fxp<+/-,64,-18>)
              n190 = Bundle(cluster=w544, "First Correlation"=w546, "Latest Correlation"=0) -> (w545:T11)
              n191 = To Fixed-Point(fixed-point type=w533, number=w541) -> (fixed-point=w534:fxp<+,32,-41>)
              n192 = Less?(x=w534, y=w533) -> (x < y?=w553:bool)
              n193 = Greater?(x=w534, y=w554) -> (0:w552:bool)
              n194 = And(x=w553, y=w552) -> (x .and. y?=w551:bool)
              n195 = case shown="True" w551 {
                tunnel: [_ u8 8 ("Det 3")] -> w550
                tunnel: [u8 9 ("Det 3") _] -> w549
                frame True {
                }
                frame False {
                }
              }
            }
            frame 9 {
              # "Wait for the particle to get to the second detector."
              n196 = Increment(x=w569) -> (x+1=w566:T10)
              n197 = Unbundle By Name(w567) -> ("Gap Max Speed Count"=w564:i32)
              n198 = Unbundle By Name(w566) -> ("Detector Gap Count"=w565:i32)
              n199 = Greater Or Equal?(x=w565, y=w564) -> (x >= y?=w563:bool)
              n200 = case shown="True" w563 {
                tunnel: [u8 10 ("State") u8 9 ("State")] -> w562
                frame True {
                }
                frame False {
                }
              }
            }
            frame 10 {
              # "Waits for a correlation that's close to the first two correlations."
              n201 = Increment(x=w591) -> (x+1=w575:T10)
              n202 = Unbundle By Name(w580) -> ("First Correlation"=w579:i32)
              n203 = Unbundle By Name(w590) -> ("Gap Min Speed Count"=w589:i32)
              n204 = Unbundle(w575) -> ("First Detector Count"=w577:i32, "Detector Gap Count"=w574:i32)  [unwired: 2 out]
              n205 = Greater Or Equal?(x=w574, y=w589) -> (x >= y?=w588:bool)
              n206 = case shown="False" w588 {
                tunnel: [_ w610] -> w581
                tunnel: [u8 10 _] -> w587
                tunnel: w586 -> [_ w609]
                tunnel: w585 -> [_ w606]
                tunnel: w579 -> [_ w596]
                tunnel: [_ w594] -> w578
                frame True {
                }
                frame False {
                  w593 = fxp<+/-,32,32> 0.0 ("fixed-point type")
                  n207 = Unbundle By Name(w606) -> ("Filter 1.Det 2"=w603:i32, "Filter 3.Det 2"=w605:i32, "Filter 4.Det 2"=w604:i32)
                  n208 = To Fixed-Point(fixed-point type=w593, number=w596) -> (fixed-point=w599:fxp<+/-,32,32>)
                  n209 = Subtract(x=fxp<+,1,2> 2.0, y=w609) -> (x-y=w607:fxp<+/-,33,17>)
                  n210 = Add(x=w605, y=w604) -> (x+y=w602:i32)
                  n211 = Multiply(x=w607, y=w599) -> (x*y=w601:fxp<+/-,64,48>)
                  n212 = Subtract(x=w602, y=w603) -> (x-y=w595:i32)
                  n213 = To Fixed-Point(fixed-point type=w593, number=w595) -> (fixed-point=w598:fxp<+/-,32,32>)
                  n214 = Greater?(x=w598, y=w601) -> (0:w600:bool)
                  n215 = case shown="True" w600 {
                    tunnel: [u8 11 u8 10] -> w610
                    frame True {
                    }
                    frame False {
                    }
                  }
                  n216 = Bundle(cluster=T11 {"First Correlation"=0, "Latest Correlation"=0} ("input cluster"), "First Correlation"=w596, "Latest Correlation"=w595) -> (w594:T11)
                }
              }
              n217 = Add(x=w584, y=w583) -> (x+y=w582:i32)
              n218 = Bundle(cluster=w575, "First Detector Count"=w577, "Detector Gap Count"=w574, "Second Detector Count"=0) -> (w576:T10)  [unwired: 1 in]
            }
            frame 11 {
              # "Searches for a maximum correlation. If the maximum correlation happens\nafter the speed limit, this isn't the right filter, and we go back to the beginning.\nIf the maximum correlation is too big, we also go back to the beginning."
              n219 = Decrement(x=w639) -> (x-1=w637:i32)
              n220 = Unbundle By Name(w630) -> ("Filter 1.Det 2"=w619:i32, "Filter 3.Det 2"=w629:i32, "Filter 4.Det 2"=w628:i32)
              n221 = Unbundle By Name(w623) -> ("Gap Min Speed Count"=w621:i32)
              n222 = Unbundle By Name(w632) -> ("Latest Correlation"=w625:i32)
              n223 = Add(x=w629, y=w628) -> (x+y=w618:i32)
              n224 = Subtract(x=w618, y=w619) -> (x-y=w631:i32)
              n225 = Increment(x=w636) -> (x+1=w624:T10)
              n226 = Add(x=w625, y=w638) -> (x+y=w626:i32)
              n227 = Greater?(x=w631, y=w626) -> (0:w634:bool)
              n228 = case shown="True" w634 {
                tunnel: [w646 w662] -> w627
                tunnel: w624 -> [w646 w659]
                tunnel: w631 -> [_ w653]
                tunnel: [w647 w661] -> w633
                tunnel: w632 -> [w647 w660]
                tunnel: [_ w650] -> w622
                tunnel: w615 -> [_ w657]
                tunnel: [_ w651] -> w614
                frame False {
                }
                frame True {
                  w649 = fxp<+/-,32,32> 0.0 ("fixed-point type")
                  n229 = Unbundle(w659) -> ("First Detector Count"=w658:i32, "Detector Gap Count"=w650:i32)  [unwired: 2 out]
                  n230 = Unbundle(w660) -> ("First Correlation"=w656:i32)  [unwired: 1 out]
                  n231 = To Fixed-Point(fixed-point type=w649, number=w656) -> (fixed-point=w655:fxp<+/-,32,32>)
                  n232 = Bundle(cluster=w660, "First Correlation"=w656, "Latest Correlation"=w653) -> (w661:T11)
                  n233 = To Fixed-Point(fixed-point type=w649, number=w653) -> (fixed-point=w652:fxp<+/-,32,32>)
                  n234 = Multiply(x=w657, y=w655) -> (x*y=w654:fxp<+/-,64,48>)
                  n235 = Bundle(cluster=w659, "First Detector Count"=w658, "Detector Gap Count"=w650, "Second Detector Count"=0) -> (w662:T10)  [unwired: 1 in]
                  n236 = Less?(x=w654, y=w652) -> (x < y?=w651:bool)
                }
              }
              n237 = Greater?(x=w622, y=w621) -> (0:w620:bool)
              n238 = Or(x=w614, y=w620) -> (x .or. y?=w616:bool)
              n239 = case shown="False" w616 {
                tunnel: w637 -> [w642 _]
                tunnel: [w641 _] -> w635
                tunnel: [_ u8 11 ("Det 3")] -> w617
                frame False {
                  n240 = Less Or Equal To 0?(x=w642) -> (x <= 0?=w640:bool)
                  n241 = case shown="True" w640 {
                    tunnel: [u8 12 ("Det 3") u8 11 ("Det 3")] -> w641
                    frame True {
                    }
                    frame False {
                    }
                  }
                }
                frame True {
                }
              }
            }
            frame 12 {
              # "Wait for the particle to get to the second detector."
              n242 = Increment(x=w671) -> (x+1=w668:T10)
              n243 = Unbundle By Name(w669) -> ("Detector Max Speed Count"=w666:i32)
              n244 = Unbundle By Name(w668) -> ("Second Detector Count"=w667:i32)
              n245 = Greater Or Equal?(x=w667, y=w666) -> (x >= y?=w665:bool)
              n246 = case shown="True" w665 {
                tunnel: [u8 13 ("State") u8 12 ("State")] -> w664
                frame True {
                }
                frame False {
                }
              }
            }
            frame 13 {
              # "Waits for a reverse correlation that's close to the first two correlations."
              n247 = Increment(x=w695) -> (x+1=w677:T10)
              n248 = Unbundle By Name(w686) -> ("First Correlation"=w685:i32)
              n249 = Unbundle By Name(w694) -> ("Detector Min Speed Count"=w693:i32)
              n250 = Unbundle By Name(w677) -> ("Second Detector Count"=w683:i32)
              n251 = Greater Or Equal?(x=w683, y=w693) -> (x >= y?=w681:bool)
              n252 = case shown="False" w681 {
                tunnel: [_ w714] -> w687
                tunnel: [u8 13 _] -> w692
                tunnel: w691 -> [_ w713]
                tunnel: w680 -> [_ w710]
                tunnel: w685 -> [_ w701]
                tunnel: [_ w699] -> w684
                frame True {
                }
                frame False {
                  w697 = fxp<+/-,32,32> 0.0 ("fixed-point type")
                  n253 = Unbundle By Name(w710) -> ("Filter 1.Det 2"=w707:i32, "Filter 3.Det 2"=w709:i32, "Filter 4.Det 2"=w708:i32)
                  n254 = To Fixed-Point(fixed-point type=w697, number=w701) -> (fixed-point=w704:fxp<+/-,32,32>)
                  n255 = Subtract(x=fxp<+,1,2> 2.0, y=w713) -> (x-y=w711:fxp<+/-,33,17>)
                  n256 = Add(x=w709, y=w708) -> (x+y=w706:i32)
                  n257 = Multiply(x=w711, y=w704) -> (x*y=w705:fxp<+/-,64,48>)
                  n258 = Subtract(x=w707, y=w706) -> (x-y=w700:i32)
                  n259 = To Fixed-Point(fixed-point type=w697, number=w700) -> (fixed-point=w703:fxp<+/-,32,32>)
                  n260 = Greater?(x=w703, y=w705) -> (0:w698:bool)
                  n261 = case shown="True" w698 {
                    tunnel: [u8 14 u8 13] -> w714
                    frame True {
                    }
                    frame False {
                    }
                  }
                  n262 = Bundle(cluster=T11 {"First Correlation"=0, "Latest Correlation"=0} ("input cluster"), "First Correlation"=w701, "Latest Correlation"=w700) -> (w699:T11)
                }
              }
              n263 = Add(x=w690, y=w689) -> (x+y=w688:i32)
              n264 = Unbundle(w677) -> ("First Detector Count"=w679:i32, "Detector Gap Count"=w676:i32, "Second Detector Count"=w675:i32)  [unwired: 1 out]
              n265 = Bundle(cluster=w677, "First Detector Count"=w679, "Detector Gap Count"=w676, "Second Detector Count"=w675, "Second Detector Final Count"=0) -> (w678:T10)
            }
            frame 14 {
              # "Searches for a maximum correlation. If the maximum correlation happens\nafter the speed limit, this isn't the right filter, and we go back to the beginning.\nIf the maximum correlation is too big, we also go back to the beginning."
              n266 = Decrement(x=w743) -> (x-1=w741:i32)
              n267 = Unbundle By Name(w734) -> ("Filter 1.Det 2"=w724:i32, "Filter 3.Det 2"=w733:i32, "Filter 4.Det 2"=w732:i32)
              n268 = Unbundle By Name(w727) -> ("Gap Min Speed Count"=w725:i32)
              n269 = Unbundle By Name(w736) -> ("Latest Correlation"=w729:i32)
              n270 = Add(x=w733, y=w732) -> (x+y=w723:i32)
              n271 = Subtract(x=w724, y=w723) -> (x-y=w735:i32)
              n272 = Increment(x=w740) -> (x+1=w728:T10)
              n273 = Add(x=w729, y=w742) -> (x+y=w730:i32)
              n274 = Greater?(x=w735, y=w730) -> (0:w738:bool)
              n275 = case shown="True" w738 {
                tunnel: [w750 w767] -> w731
                tunnel: w728 -> [w750 w764]
                tunnel: w735 -> [_ w758]
                tunnel: [w751 w766] -> w737
                tunnel: w736 -> [w751 w765]
                tunnel: [_ w754] -> w726
                tunnel: w720 -> [_ w762]
                tunnel: [_ w756] -> w719
                frame False {
                }
                frame True {
                  w753 = fxp<+/-,32,32> 0.0 ("fixed-point type")
                  n276 = Unbundle(w764) -> ("First Detector Count"=w763:i32, "Detector Gap Count"=w755:i32, "Second Detector Count"=w754:i32)  [unwired: 1 out]
                  n277 = Unbundle(w765) -> ("First Correlation"=w761:i32)  [unwired: 1 out]
                  n278 = Bundle(cluster=w764, "First Detector Count"=w763, "Detector Gap Count"=w755, "Second Detector Count"=w754, "Second Detector Final Count"=0) -> (w767:T10)
                  n279 = To Fixed-Point(fixed-point type=w753, number=w761) -> (fixed-point=w760:fxp<+/-,32,32>)
                  n280 = Bundle(cluster=w765, "First Correlation"=w761, "Latest Correlation"=w758) -> (w766:T11)
                  n281 = To Fixed-Point(fixed-point type=w753, number=w758) -> (fixed-point=w757:fxp<+/-,32,32>)
                  n282 = Multiply(x=w762, y=w760) -> (x*y=w759:fxp<+/-,64,48>)
                  n283 = Less?(x=w759, y=w757) -> (x < y?=w756:bool)
                }
              }
              n284 = Greater?(x=w726, y=w725) -> (0:w717:bool)
              n285 = And(x=w719, y=w717) -> (x .and. y?=w721:bool)
              n286 = case shown="False" w721 {
                tunnel: w741 -> [w746 _]
                tunnel: [w745 _] -> w739
                tunnel: [_ u8 14 ("Det 3")] -> w722
                frame False {
                  n287 = Less Or Equal To 0?(x=w746) -> (x <= 0?=w744:bool)
                  n288 = case shown="False" w744 {
                    tunnel: [u8 15 ("Det 3") u8 14 ("Det 3")] -> w745
                    frame True {
                    }
                    frame False {
                    }
                  }
                }
                frame True {
                }
              }
            }
            frame 15 {
              # "v = clockspeed * distance / speed count"
              # "1/2mv^2 = Vq\ntherefore\nm = 2Vq/v^2"
              n289 = Increment(x=w801) -> (x+1=w800:T10)
              n290 = Unbundle By Name(w802) -> ("High Velocity Limit"=w782:fxp<+,18,18>, "Low Velocity Limit"=w783:fxp<+,18,18>, "High Mass Limit"=w792:fxp<+/-,33,-36>, "Low Mass Limit"=w793:fxp<+/-,33,-36>, "High Voltage"=w787:fxp<+,16,22>)
              n291 = Unbundle By Name(w800) -> ("First Detector Count"=w799:i32, "Second Detector Final Count"=w798:i32)
              n292 = Multiply(x=w787, y=w768) -> (x*y=w794:fxp<+,48,-19>)
              n293 = Subtract(x=w799, y=w798) -> (x-y=w769:i32)
              n294 = To Fixed-Point(fixed-point type=fxp<+/-,32,32> 0.0, number=w769) -> (fixed-point=w781:fxp<+/-,32,32>)
              n295 = To Fixed-Point(fixed-point type=fxp<+,21,21> 0.0, number=w769) -> (fixed-point=w770:fxp<+,21,21>)
              n296 = Square(x=w770) -> (x^2=w771:fxp<+,42,42>)
              n297 = Multiply(x=w782, y=w781) -> (x*y=w780:fxp<+/-,50,50>)
              n298 = Multiply(x=w781, y=w783) -> (x*y=w779:fxp<+/-,50,50>)
              n299 = Multiply(x=w796, y=w771) -> (x*y=w795:fxp<+/-,64,0>)
              n300 = Multiply(x=w794, y=w795) -> (x*y=w772:fxp<+/-,64,-19>)
              n301 = Greater Or Equal?(x=w780, y=w778) -> (x >= y?=w791:bool)
              n302 = Less Or Equal?(x=w779, y=w778) -> (x <= y?=w790:bool)
              n303 = Scale By Power Of 2(n=i16 1, x=w772) -> (x*2^n=w773:fxp<+/-,64,-19>)
              n304 = Less Or Equal?(x=w773, y=w792) -> (x <= y?=w789:bool)
              n305 = Greater Or Equal?(x=w773, y=w793) -> (x >= y?=w788:bool)
              n306 = Compound Arithmetic op=AND(w791, w790, w789, w788, w777) -> (w776:bool)
              n307 = case shown="True" w776 {
                tunnel: [u8 16 ("Det 3") _] -> w785
                tunnel: [_ u8 15 ("Det 3")] -> w784
                frame True {
                }
                frame False {
                }
              }
            }
            frame 16 {
              n308 = Increment(x=w821) -> (x+1=w820:T10)
              n309 = Unbundle By Name(w820) -> ("First Detector Count"=w819:i32, "Second Detector Final Count"=w810:i32)
              n310 = Subtract(x=w819, y=w810) -> (x-y=w816:i32)
              n311 = To Fixed-Point(fixed-point type=fxp<+/-,32,32> 0.0, number=w816) -> (fixed-point=w818:fxp<+/-,32,32>)
              n312 = Multiply(x=w818, y=w817) -> (x*y=w815:T14)
              n313 = To Long Integer(number=w815) -> (32bit integer=w814:T15)
              n314 = Subtract(x=w814, y=w813) -> (x-y=w812:T15)
              n315 = Subtract(x=w812, y=w810) -> (x-y=w809:T15)
              n316 = Unbundle By Name(w809) -> ("Distance to DCS 1"=w807:i32)
              n317 = Add(x=w807, y=w808) -> (x+y=w806:i32)
            }
            frame 17 {
              n318 = Decrement(x=w826) -> (x-1=w825:T15)
              n319 = Unbundle By Name(w825) -> ("Distance to PSU"=w824:i32)
              n320 = Less Or Equal To 0?(x=w824) -> (x <= 0?=w822:bool)
              n321 = case shown="True" w822 {
                tunnel: [u8 18 ("Det 3") u8 17 ("Det 3")] -> w823
                frame True {
                }
                frame False {
                }
              }
            }
            frame 18 {
              n322 = Decrement(x=w834) -> (x-1=w833:T15)
              n323 = Unbundle By Name(w833) -> ("Distance to end of PSU"=w832:i32)
              n324 = Less Or Equal To 0?(x=w832) -> (x <= 0?=w830:bool)
              n325 = case shown="True" w830 {
                tunnel: [u8 19 ("Det 3") u8 18 ("Det 3")] -> w831
                frame True {
                }
                frame False {
                }
              }
            }
            frame 19 {
              n326 = Decrement(x=w841) -> (x-1=w840:T15)
              n327 = Unbundle By Name(w840) -> ("Distance to DCS 2"=w839:i32)
              n328 = Less Or Equal To 0?(x=w839) -> (x <= 0?=w837:bool)
              n329 = case shown="True" w837 {
                tunnel: [u8 20 ("Det 3") u8 19 ("Det 3")] -> w838
                frame True {
                }
                frame False {
                }
              }
            }
            frame 20 {
              n330 = Decrement(x=w850) -> (x-1=w849:T15)
              n331 = Unbundle By Name(w849) -> ("Distance to DCS 2"=w848:i32)
              n332 = Add(x=w848, y=w847) -> (x+y=w846:i32)
              n333 = Less Or Equal To 0?(x=w846) -> (x <= 0?=w845:bool)
              n334 = case shown="True" w845 {
                tunnel: [u8 20 ("Det 3") w855] -> w852
                tunnel: w844 -> [_ w854]
                frame False {
                }
                frame True {
                  n335 = case shown="True" w854 {
                    tunnel: [_ u8 21 ("Det 3")] -> w855
                    frame False {
                    }
                    frame True {
                    }
                  }
                }
              }
            }
            frame 21 {
              n336 = Decrement(x=w861) -> (x-1=w860:T15)
              n337 = Unbundle By Name(w860) -> ("Distance to front of LEIL Chamber"=w859:i32)
              n338 = Less Or Equal To 0?(x=w859) -> (x <= 0?=w857:bool)
              n339 = case shown="True" w857 {
                tunnel: [u8 22 ("Det 3") u8 21 ("Det 3")] -> w858
                frame True {
                }
                frame False {
                }
              }
            }
            frame 22 {
              n340 = Decrement(x=w870) -> (x-1=w869:T15)
              n341 = Unbundle By Name(w869) -> ("Distance to front of LEIL Chamber"=w868:i32)
              n342 = Add(x=w868, y=w867) -> (x+y=w866:i32)
              n343 = Less Or Equal To 0?(x=w866) -> (x <= 0?=w865:bool)
              n344 = case shown="False" w865 {
                tunnel: [u8 22 ("Det 3") _] -> w871
                frame False {
                }
                frame True {
                }
              }
            }
          }
        }
      }
      n345 = disable-structure shown="Disabled" {
        disable-tunnel: w240 -> [w888 w896]
        disable-tunnel: [w884 w895] -> w236
        disable-tunnel: [w886 _] -> w235
        disable-tunnel: w234 -> [w887 _]
        frame Disabled {
          n346 = case shown="1, Default" w888 {
            selector: w888 -> [_ w894]
            tunnel: [w891 w892] -> w885
            tunnel: w887 -> [w891 w893]
            frame 0 {
            }
            frame 1, Default {
              n347 = Max & Min(x=w894, y=w893) -> (min(x,y)=w892:i32)  [unwired: 1 out]
            }
          }
          n348 = Less Than 0?(x=w885) -> (x < 0?=w884:bool)
          n349 = case shown="False" w884 {
            tunnel: w885 -> [w890 _]
            tunnel: [w889 _] -> w886
            frame False {
              n350 = Decrement(x=w890) -> (x-1=w889:i32)
            }
            frame True {
            }
          }
        }
        frame Enabled {
          n351 = Not Equal To 0?(x=w896) -> (x != 0?=w895:bool)
        }
      }
      n352 = case shown="True" w218 {
        tunnel: w229 -> [_ w875]
        tunnel: w228 -> [_ w876]
        tunnel: w227 -> [_ w877]
        tunnel: [w873 w874] -> w215
        tunnel: w216 -> [w873 _]
        frame False {
        }
        frame True {
          n353 = Bundle(w877, w876, "High Charge Limit"=w875) -> (w874:T16)  [unwired: 1 in]
        }
      }
      n354 = case shown="False" w236 {
        tunnel: w239 -> [_ w883]
        tunnel: [w878 w883] -> w238
        tunnel: w237 -> [w879 _]
        frame False {
          n355 = case shown="1, Default" w879 {
            selector: w879 -> [w880 w882]
            tunnel: [w880 w881] -> w878
            frame 0 {
            }
            frame 1, Default {
              n356 = Decrement(x=w882) -> (x-1=w881:u16)
            }
          }
        }
        frame True {
        }
      }
      n357 = Unbundle(w215) -> (w214:i32, w213:fxp<+/-,64,-19>, "High Charge Limit"=w212:fxp<+,32,-41>)
    }
    "Velocity Count" <- w105
    "Mass" <- w104
    "Charge" <- w103
    n358 = case shown="False" "Calibrate" {
      tunnel: w143 -> [w198 _]
      tunnel: w108 -> [w199 w202]
      tunnel: [w199 w200] -> w165
      tunnel: w142 -> [_ w201]
      tunnel: [w198 _] -> w102
      tunnel: w101 -> [_ _]
      frame False {
      }
      frame True {
        n359 = for {
          tunnel: w201 -> [w205] mode=indexing
          tunnel: w202 -> [w204] mode=indexing
          tunnel: [w203] -> w200 mode=indexing
          n360 = Max & Min(x=w204, y=w205) -> (max(x,y)=w203:i32)  [unwired: 1 out]
        }
      }
    }
    n361 = Or Array Elements(Boolean array=w124) -> (logical OR=w118:bool)
    n362 = Not(x=w118) -> (.not. x?=w123:bool)
    n363 = Or Array Elements(Boolean array=w129) -> (logical OR=w115:bool)
    "Plates" <- w115
    n364 = Or Array Elements(Boolean array=w128) -> (logical OR=→"DCS 2":bool)
    n365 = Or Array Elements(Boolean array=w127) -> (logical OR=→"User Trigger":bool)
    n366 = Greater Than 0?(x=w159) -> (x > 0?=w139:bool[])
    n367 = And(x=w123, y=w121) -> (x .and. y?=w122:bool)
    n368 = Or Array Elements(Boolean array=w139) -> (logical OR=→"DCS 1":bool)
    n369 = local write "Armed"(w122) -> ()
  }
  "PSU Response" <- w9
  "Thresholds out" <- w24
  n370 = Array Max & Min(array=w8) -> (max value=w4:u8, max index (indices)=w7:i32[])  [unwired: 2 out]
  n371 = local read "Max Stop Point"() -> (w2:T1)
  n372 = Index Array(array=w7) -> (element #1=w5:i32, element #2=w6:i32)  [unwired: 2 in]
  n373 = Bundle(cluster=w2, "Max Stop"=w4, "Index"=w5, "Filter"=w6) -> (→"Max Stop Point":T1)
